vi "ATM Messages (SubVI).vi"(7 "Message Type":T1, 8 "error in (no error)":errorcluster, 10 "replace string (\"\")":string="Thomas Klinger", 11 "search string":string="<NAME>") -> (0 "error out":errorcluster, 3 "Message out":string)   [LabVIEW 2018]
uses:
  Controls/Messages.ctl
panel:
  # "Input Values"
  # "Output Values"
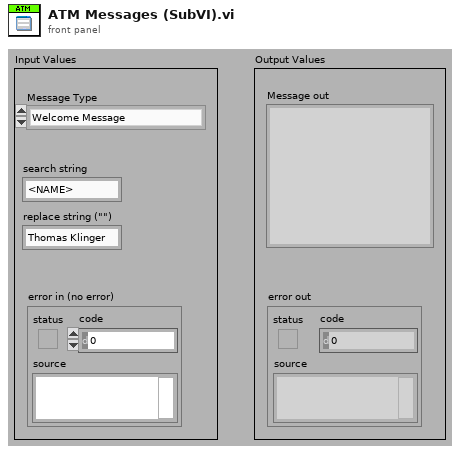
[diagram p1: front panel]
types:
  T1 = typedef "Messages.ctl" = enum16{"Welcome Message", "Main Menu Message", "Account Verification Failed Message", "Session Terminate Message", "Deposit Message", "Deposit Complete Message", "Withdrawal Message", "Withdrawal Complete Message", "Withdrawal Failed Message", "Balance Inquiry Message"}
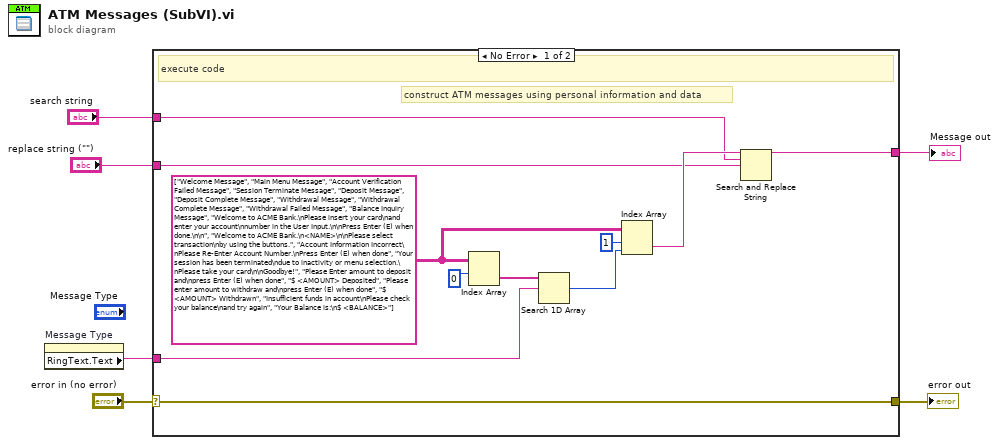
[diagram p0: block diagram]
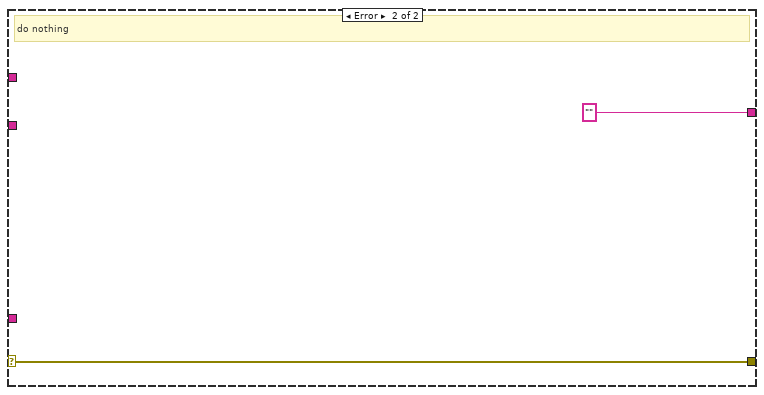
[diagram p2: hidden frame]
diagram:
  n1 = property on="Message Type" class="Enum (strict)"() -> ("RingText.Text"=w3:string)  [unwired: 2 in, 2 out]
  n2 = case shown="No Error" "error in (no error)" {
    selector: "error in (no error)" -> [w9 w19]
    tunnel: w3 -> [w11 _]
    tunnel: [w10 "" ("result string")] -> w6
    tunnel: [w9 w19] -> w4
    tunnel: "search string" -> [w8 _]
    tunnel: "replace string (\"\")" -> [w7 _]
    frame No Error {
      w15 = string[][] [["Welcome Message", "Main Menu Message", "Account Verification Failed Message", "Session Terminate Message", "Deposit Message", "Deposit Complete Message", "Withdrawal Message", "Withdrawal Complete Message", "Withdrawal Failed Message", "Balance Inquiry Message"], ["Welcome to ACME Bank.\nPlease insert your card\nand enter your account\nnumber in the User Input.\n\nPress Enter (E) when done.\n\n", "Welcome to ACME Bank.\n<NAME>\n\nPlease select transaction\nby using the buttons.", "Account Information Incorrect\nPlease Re-Enter Account Number.\nPress Enter (E) when done", "Your session has been terminated\ndue to inactivity or menu selection.\nPlease take your card\n\nGoodbye!", "Please Enter amount to deposit and\npress Enter (E) when done", "$ <AMOUNT> Deposited", "Please enter amount to withdraw and\npress Enter (E) when done", "$ <AMOUNT> Withdrawn", "Insufficient funds in account\nPlease check your balance\nand try again", "Your Balance is:\n$ <BALANCE>"]]
      # "construct ATM messages using personal information and data"
      # "execute code"
      n3 = Index Array "Index Array"(array=w15, index (row)=0) -> (element=w16:string[])  [unwired: 1 in]
      n4 = Search 1D Array(1D array=w16, element=w11) -> (index of element=w13:i32)  [unwired: 1 in]
      n5 = Index Array "Index Array"(array=w15, index (row)=1, index (col)=w13) -> (element=w12:string)
      n6 = Search and Replace String(input string=w12, search string=w8, replace string=w7) -> (result string=w10:string)  [unwired: 5 in, 3 out]
    }
    frame Error {
      # "do nothing"
    }
  }
  "Message out" <- w6
  "error out" <- w4
